vi "Data.Build Result Attribute.vi"(4 "Desc":string, 6 "Code":i32, 7 "Category":string, 8 "Error":errorcluster, 9 "Status":T1 caption="Status (Log)" items=["LOG", "PASS", "FAIL", "ERROR"], 10 "Value":string, 11 "Name":string) -> (3 "Attribute":T2 {"Status" items=["LOG", "PASS", "FAIL", "ERROR"]})   [LabVIEW 2024, in "EQMF.lvlib" / "Data.lvlib"]
uses:
  Data.lvlib
  TypeDefs/Data.Result Attribute.ctl
  TypeDefs/Data.Result Item Status.ctl
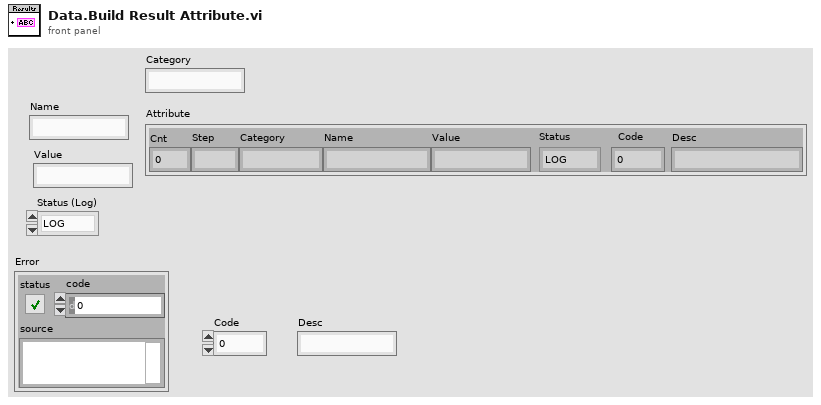
[diagram p1: front panel]
types:
  T1 = typedef "EQMF.lvlib/Data.lvlib/Data.Result Item Status.ctl" = i32
  T2 = typedef "EQMF.lvlib/Data.lvlib/Data.Result Attribute.ctl" = cluster{"Cnt":i32, "Step":string, "Category":string, "Name":string, "Value":string, "Status":T1, "Code":i32, "Desc":string}
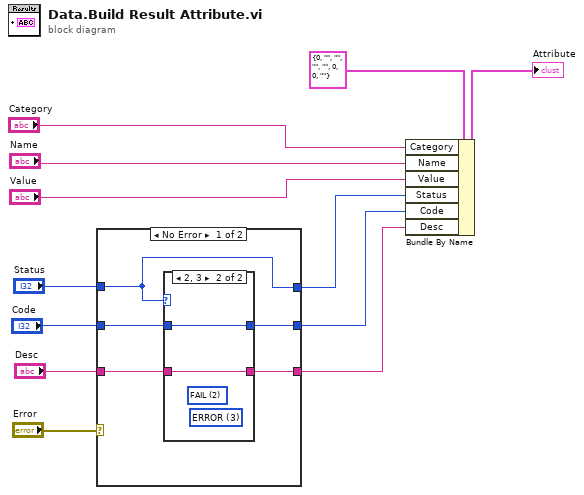
[diagram p0: block diagram]
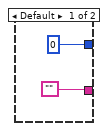
[diagram p2: hidden frame]
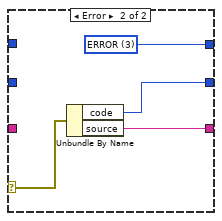
[diagram p3: hidden frame]
diagram:
  n1 = case shown="No Error" "Error" {
    selector: "Error" -> [_ w25]
    tunnel: "Status" -> [w13 _]
    tunnel: [w17 w24] -> w6
    tunnel: "Code" -> [w16 _]
    tunnel: "Desc" -> [w15 _]
    tunnel: [w14 w23] -> w3
    tunnel: [w13 w22] -> w1
    frame No Error {
      n2 = case shown="2, 3" w13 {
        tunnel: [0 w21] -> w17
        tunnel: w16 -> [_ w21]
        tunnel: w15 -> [_ w20]
        tunnel: ["" w20] -> w14
        frame Default {
        }
        frame 2, 3 {
          (unwired) T1 3 items=["LOG", "PASS", "FAIL", "ERROR"] ("Status")
          (unwired) T1 2 items=["LOG", "PASS", "FAIL", "ERROR"] ("Status")
        }
      }
    }
    frame Error {
      w22 = T1 3 items=["LOG", "PASS", "FAIL", "ERROR"] ("Status")
      n3 = Unbundle By Name(w25) -> ("code"=w24:i32, "source"=w23:string)
    }
  }
  n4 = Bundle By Name(cluster=T2 {"Cnt"=0, "Step"="", "Category"="", "Name"="", "Value"="", "Status"=0, "Code"=0, "Desc"=""} ("Attribute"), "Category"="Category", "Name"="Name", "Value"="Value", "Status"=w1, "Code"=w6, "Desc"=w3) -> (→"Attribute":T2)
